vi "Get Channel Stats.vi"(8 "Array Length":i32, 9 "Number of Precision Digits":i32, 10 "Log Stats":bool, 11 "TDMS Channel Info":T1) -> (3 "Channel Stats":string[](array[string]))   [LabVIEW 2022 SP3, in "CSV Export.lvlib" / "CSV Export.lvclass"]
uses:
  CSV Export.lvclass
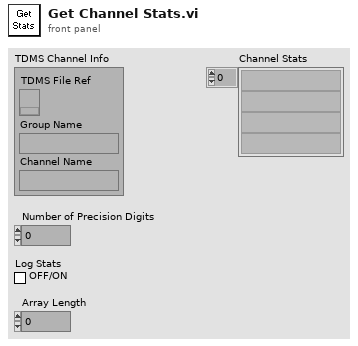
[diagram p1: front panel]
types:
  T1 = cluster{"TDMS File Ref":refnum<k34>, "Group Name":string, "Channel Name":string}
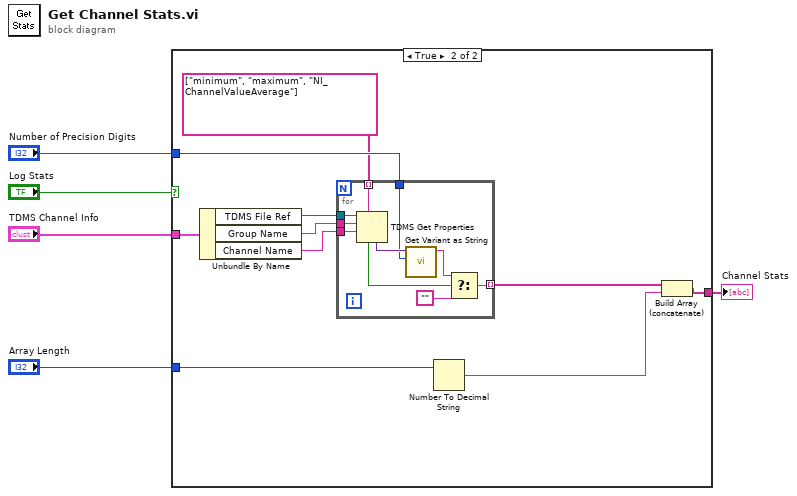
[diagram p0: block diagram]
diagram:
  n1 = case shown="True" "Log Stats" {
    tunnel: "TDMS Channel Info" -> [_ w14]
    tunnel: "Number of Precision Digits" -> [_ w10]
    tunnel: [_ w15] -> w3
    tunnel: "Array Length" -> [_ w6]
    frame False {
    }
    frame True {
      n2 = Unbundle By Name(w14) -> ("TDMS File Ref"=w13:refnum<k34>, "Group Name"=w12:string, "Channel Name"=w11:string)
      n3 = for {
        tunnel: w13 -> [w25]
        tunnel: w12 -> [w24]
        tunnel: w11 -> [w23]
        tunnel: w10 -> [w21]
        tunnel: string[] ["minimum", "maximum", "NI_ChannelValueAverage"] -> [w20] mode=indexing
        tunnel: [w16] -> w8 mode=indexing
        n4 = TDMS Get Properties(7:w20, 9:w23, 10:w24, 11:w25) -> (4:w22:variant, 6:w19:bool)  [unwired: 2 in, 4 out]
        n5 = call "Get Variant as String.vi"("Digits of Precision"=w21, "Variant"=w22) -> ("Variant Value as String"=w18:string)  [unwired: 9 in]
        n6 = Select(t=w18, s=w19, f="") -> (s? t:f=w16:string)
      }
      n7 = Number To Decimal String(number=w6) -> (decimal integer string=w7:string)  [unwired: 1 in]
      n8 = Build Array (concatenate)(w8, w7) -> (w15:string[])
    }
  }
  "Channel Stats" <- w3
